vi "_Match String Inside Pattern.vi"(7 "Cluster":cluster{"left":string, "right":string}={"left"="(", "right"=")"}, 11 "string":string) -> (3 "String inside":string)   [LabVIEW 2017, in "CSM_ExampleBrowser.lvlib"]
uses:
  CSM_ExampleBrowser.lvlib
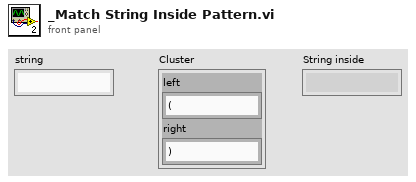
[diagram p1: front panel]
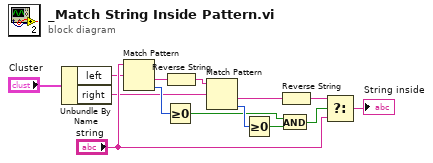
[diagram p0: block diagram]
diagram:
  n1 = Unbundle By Name("Cluster") -> ("left"=w5:string, "right"=w4:string)
  n2 = Match Pattern(string="string", regular expression=w5) -> (after substring=w14:string, offset past match=w12:i32)  [unwired: 1 in, 2 out]
  n3 = Greater Or Equal To 0?(x=w12) -> (x >= 0?=w11:bool)
  n4 = Reverse String(1:w14) -> (0:w3:string)
  n5 = Match Pattern(string=w3, regular expression=w4) -> (after substring=w2:string, offset past match=w13:i32)  [unwired: 1 in, 2 out]
  n6 = Greater Or Equal To 0?(x=w13) -> (x >= 0?=w10:bool)
  n7 = And(x=w11, y=w10) -> (x .and. y?=w9:bool)
  n8 = Reverse String(1:w2) -> (0:w1:string)
  n9 = Select(t=w1, s=w9, f="string") -> (s? t:f=→"String inside":string)
